vi "Draw Border.vi"(8 "error in (no error)":errorcluster, 11 "Line Border in":refnum<class "Line Border.lvclass">) -> (0 "error out":errorcluster, 2 "Border out":picture, 3 "Line Border out":refnum<class "Line Border.lvclass">)   [LabVIEW 2015, in "Line Border.lvclass"]
uses:
  Line Border.lvclass
  Line Border.lvclass/Line Border.ctl
  Scalable Border/Scalable Border.lvclass/Scalable Border.ctl
  Scalable Border/Scalable Border.lvclass
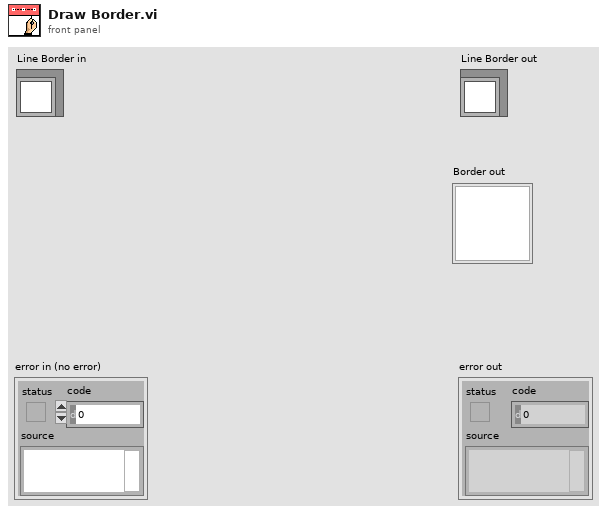
[diagram p1: front panel]
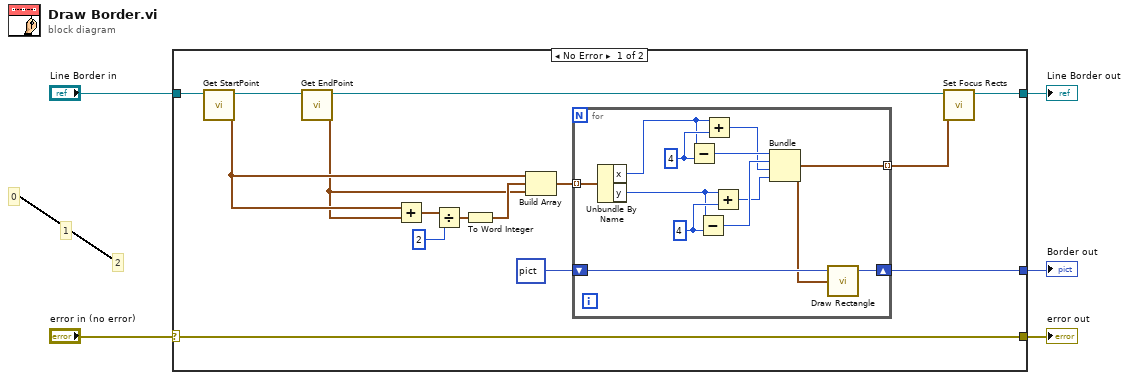
[diagram p0: block diagram]
diagram:
  # "2"
  # "1"
  # "0"
  n1 = case shown="No Error" "error in (no error)" {
    selector: "error in (no error)" -> [w20 w34]
    tunnel: "Line Border in" -> [w19 w33]
    tunnel: [w7 w33] -> w3
    tunnel: [w9 _] -> w2
    tunnel: [w20 w34] -> w1
    frame No Error {
      n2 = call "Get StartPoint.vi"("Line Border in"=w19) -> ("StartPoint"=w13:cluster{"x":i16, "y":i16}, "Line Border out"=w18:refnum<class "Line Border.lvclass">)  [unwired: 8 in, 1 out]
      n3 = call "Get EndPoint.vi"("Line Border in"=w18) -> ("EndPoint"=w11:cluster{"x":i16, "y":i16}, "Line Border out"=w17:refnum<class "Line Border.lvclass">)  [unwired: 8 in, 1 out]
      n4 = Add(x=w13, y=w11) -> (x+y=w16:cluster{"x":i16, "y":i16})
      n5 = Divide(x=w16, y=i16 2) -> (x/y=w14:cluster{"x":dbl, "y":dbl})
      n6 = To Word Integer(number=w14) -> (16bit integer=w12:cluster{"x":i16, "y":i16})
      n7 = Build Array(w13, w12, w11) -> (w10:cluster{"x":i16, "y":i16}[])
      n8 = for {
        shift-right: [w25] -> w9
        shift-left: picture data[5B] ("new picture") -> [w32]
        tunnel: w10 -> [w24] mode=indexing
        tunnel: [w21] -> w6 mode=indexing
        w30 = i16 4 ("y")
        w31 = i16 4 ("y")
        n9 = Unbundle By Name(w24) -> ("x"=w23:i16, "y"=w22:i16)
        n10 = Subtract(x=w23, y=w31) -> (x-y=w29:i16)
        n11 = Subtract(x=w22, y=w30) -> (x-y=w28:i16)
        n12 = Add(x=w23, y=w31) -> (x+y=w27:i16)
        n13 = Add(x=w22, y=w30) -> (x+y=w26:i16)
        n14 = Bundle(w29, w28, w27, w26) -> (w21:cluster{i16, i16, i16, i16})  [unwired: 1 in]
        n15 = call <vilib>:"Draw Rectangle.vi"("picture"=w32, "rect"=w21) -> ("new picture"=w25:picture)  [unwired: 7 in]
      }
      n16 = call "Set Focus Rects.vi"("Focus Rects"=w6, "Scalable Border in"=w17) -> ("Scalable Border out"=w7:refnum<class "Line Border.lvclass">)  [unwired: 8 in, 1 out]
    }
    frame Error {
    }
  }
  "error out" <- w1
  "Line Border out" <- w3
  "Border out" <- w2
